vi "pulses2commands.vi"(4 "N_pulses":i32=1 min=1, 6 "running_mode":enum16{"Continuous", "Single", "N pulses"}(ring), 8 "read_width_us":dbl=0.3, 9 "read_delay_us":dbl, 10 "pulse_width_us":dbl=50.0 format="%#.3f", 11 "pulse_period_us":dbl=100.0 format="%#_6p") -> (0 "error_out":errorcluster, 3 "instructions_array":T1(array[cluster]) {"Time" format="%#_6e"})   [LabVIEW 2018]
panel:
  # "Laser Pulse"
  # "Counting pulse"
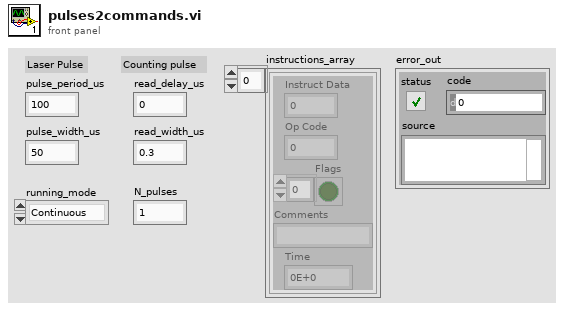
[diagram p1: front panel]
types:
  T1 = cluster{"Instruct Data":i32, "Op Code":i32, "Flags":bool[], "Comments":string, "Time":dbl}[]
  T2 = cluster{"Instruct Data":i32, "Op Code":i32, "Flags":bool[], "Comments":string, "Time":dbl}
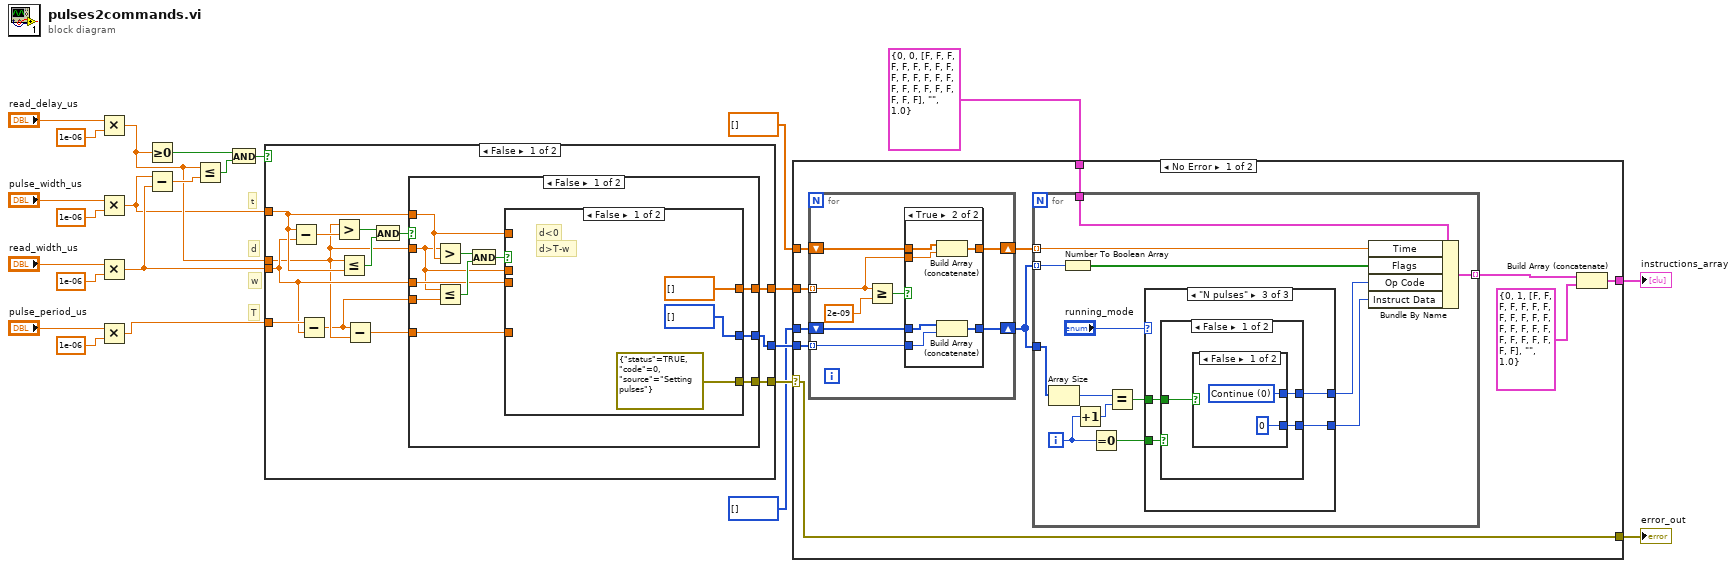
[diagram p0: block diagram]
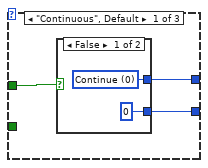
[diagram p2: hidden frame]
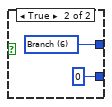
[diagram p3: hidden frame]
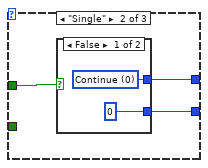
[diagram p4: hidden frame]
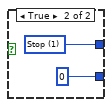
[diagram p5: hidden frame]
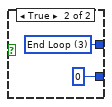
[diagram p6: hidden frame]
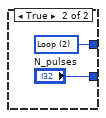
[diagram p7: hidden frame]
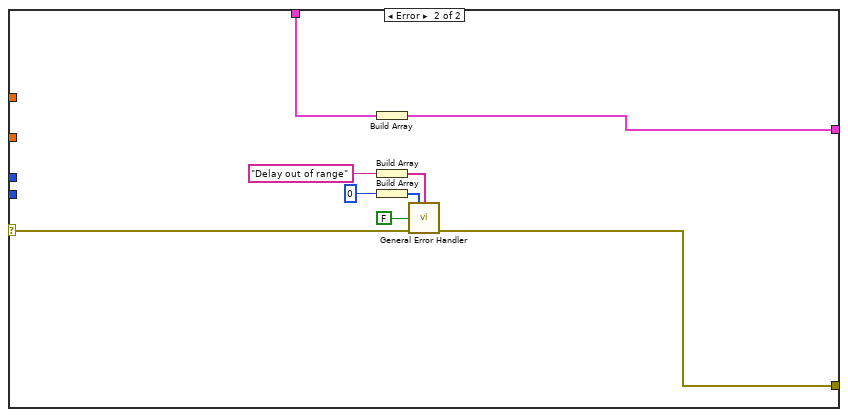
[diagram p9: hidden frame]
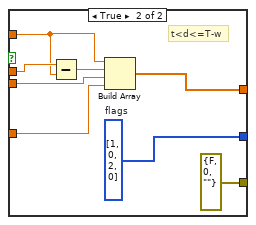
[diagram p10: hidden frame]
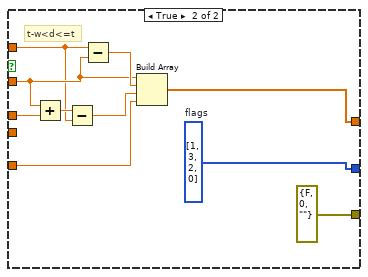
[diagram p11: hidden frame]
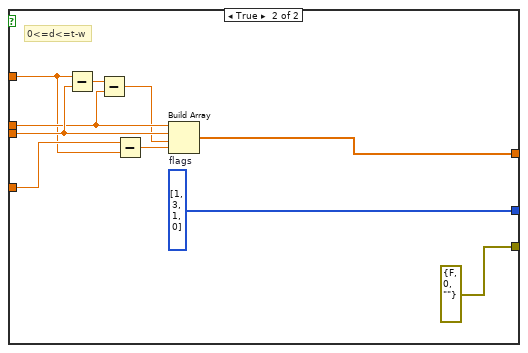
[diagram p12: hidden frame]
diagram:
  # "T"
  # "d"
  # "w"
  # "t"
  n1 = Multiply(x="read_delay_us", y=1e-06) -> (x*y=w12:dbl)
  n2 = Multiply(x="pulse_width_us", y=1e-06) -> (x*y=w4:dbl)
  n3 = Multiply(x="read_width_us", y=1e-06) -> (x*y=w16:dbl)
  n4 = Multiply(x="pulse_period_us", y=1e-06) -> (x*y=w1:dbl)
  n5 = Greater Or Equal To 0?(x=w12) -> (x >= 0?=w22:bool)
  n6 = Subtract(x=w4, y=w16) -> (x-y=w24:dbl)
  n7 = Less Or Equal?(x=w12, y=w24) -> (x <= y?=w23:bool)
  n8 = And(x=w22, y=w23) -> (x .and. y?=w21:bool)
  n9 = case shown="False" w21 {
    tunnel: w12 -> [w28 w77]
    tunnel: w16 -> [w29 w78]
    tunnel: w4 -> [w32 w70]
    tunnel: w1 -> [w33 w71]
    tunnel: [w30 w74] -> w19
    tunnel: [w26 w73] -> w20
    tunnel: [w25 errorcluster {"status"=FALSE, "code"=0, "source"=""} ("error constant")] -> w18
    frame False {
      n10 = Subtract(x=w32, y=w29) -> (x-y=w37:dbl)
      n11 = Subtract(x=w33, y=w29) -> (x-y=w27:dbl)
      n12 = Greater?(x=w28, y=w37) -> (0:w35:bool)
      n13 = Less Or Equal?(x=w28, y=w32) -> (x <= y?=w36:bool)
      n14 = Subtract(x=w27, y=w28) -> (x-y=w31:dbl)
      n15 = And(x=w35, y=w36) -> (x .and. y?=w34:bool)
      n16 = case shown="False" w34 {
        tunnel: w28 -> [w41 w68]
        tunnel: w32 -> [w44 w65]
        tunnel: w29 -> [w42 w67]
        tunnel: w31 -> [w43 w63]
        tunnel: [w40 w62] -> w30
        tunnel: w27 -> [w48 _]
        tunnel: [w39 w61] -> w26
        tunnel: [w38 errorcluster {"status"=FALSE, "code"=0, "source"=""} ("error constant")] -> w25
        frame False {
          n17 = Greater?(x=w41, y=w44) -> (0:w46:bool)
          n18 = Less Or Equal?(x=w41, y=w48) -> (x <= y?=w47:bool)
          n19 = And(x=w46, y=w47) -> (x .and. y?=w45:bool)
          n20 = case shown="False" w45 {
            tunnel: w44 -> [_ w55]
            tunnel: w43 -> [_ w59]
            tunnel: w42 -> [_ w58]
            tunnel: w41 -> [_ w56]
            tunnel: [dbl[] [] w54] -> w40
            tunnel: [u8[] [] ("flags") w53] -> w39
            tunnel: [errorcluster {"status"=TRUE, "code"=0, "source"="Setting pulses"} ("error constant") errorcluster {"status"=FALSE, "code"=0, "source"=""} ("error constant")] -> w38
            frame False {
              # "d>T-w"
              # "d<0"
            }
            frame True {
              w53 = u8[] [1, 0, 2, 0]  # flags
              # "t<d<=T-w"
              n21 = Subtract(x=w56, y=w55) -> (x-y=w57:dbl)
              n22 = Build Array(w55, w57, w58, w59) -> (w54:dbl[])
            }
          }
        }
        frame True {
          w61 = u8[] [1, 3, 2, 0]  # flags
          # "t-w<d<=t"
          n23 = Add(x=w68, y=w67) -> (x+y=w66:dbl)
          n24 = Subtract(x=w66, y=w65) -> (x-y=w64:dbl)
          n25 = Subtract(x=w65, y=w68) -> (x-y=w69:dbl)
          n26 = Build Array(w68, w69, w64, w63) -> (w62:dbl[])
        }
      }
    }
    frame True {
      w73 = u8[] [1, 3, 1, 0]  # flags
      # "0<=d<=t-w"
      n27 = Subtract(x=w70, y=w78) -> (x-y=w79:dbl)
      n28 = Subtract(x=w79, y=w77) -> (x-y=w76:dbl)
      n29 = Subtract(x=w71, y=w70) -> (x-y=w75:dbl)
      n30 = Build Array(w77, w78, w76, w75) -> (w74:dbl[])
    }
  }
  n31 = case shown="No Error" w18 {
    selector: w18 -> [w86 w154]
    tunnel: w20 -> [w84 _]
    tunnel: w19 -> [w88 _]
    tunnel: [w81 w156] -> w11
    tunnel: T2 {"Instruct Data"=0, "Op Code"=0, "Flags"=[FALSE, FALSE, FALSE, FALSE, FALSE, FALSE, FALSE, FALSE, FALSE, FALSE, FALSE, FALSE, FALSE, FALSE, FALSE, FALSE, FALSE, FALSE, FALSE, FALSE, FALSE, FALSE, FALSE, FALSE], "Comments"="", "Time"=1.0} ("PB Instruction") -> [w87 w155]
    tunnel: [w86 w153] -> w9
    tunnel: dbl[] [] ("appended array") -> [w85 _]
    tunnel: u8[] [] ("appended array") -> [w83 _]
    frame No Error {
      n32 = for {
        shift-right: [w136] -> w89
        shift-left: w83 -> [w138]
        shift-right: [w137] -> w90
        shift-left: w85 -> [w139]
        tunnel: w88 -> [w133] mode=indexing
        tunnel: w84 -> [w132] mode=indexing
        n33 = Greater Or Equal?(x=w133, y=2e-09) -> (x >= y?=w135:bool)
        n34 = case shown="True" w135 {
          tunnel: w139 -> [w140 w147]
          tunnel: w138 -> [w141 w143]
          tunnel: [w140 w146] -> w137
          tunnel: [w141 w144] -> w136
          tunnel: w133 -> [_ w145]
          tunnel: w132 -> [_ w142]
          frame False {
          }
          frame True {
            n35 = Build Array (concatenate)(w147, w145) -> (w146:dbl[])
            n36 = Build Array (concatenate)(w143, w142) -> (w144:u8[])
          }
        }
      }
      n37 = for {
        tunnel: w90 -> [w104] mode=indexing
        tunnel: w89 -> [w103] mode=indexing
        tunnel: [w97] -> w82 mode=indexing
        tunnel: w89 -> [w98]
        tunnel: w87 -> [w101]
        i -> [w95]
        n38 = Array Size(array=w98) -> (size(s)=w99:i32)
        n39 = Number To Boolean Array(number=w103) -> (Boolean array=w102:bool[])
        n40 = Increment(x=w95) -> (x+1=w100:i32)
        n41 = Equal To 0?(x=w95) -> (x = 0?=w93:bool)
        n42 = Equal?(x=w99, y=w100) -> (x = y?=w94:bool)
        n43 = case shown="\"N pulses\"" "running_mode" {
          tunnel: w94 -> [w105 w112 w122]
          tunnel: [w107 w114 w121] -> w92
          tunnel: [w106 w113 w120] -> w91
          tunnel: w93 -> [_ _ w119]
          frame "Continuous", Default {
            n44 = case shown="False" w105 {
              tunnel: [w109 w111] -> w107
              tunnel: [0 ("N_pulses") 0 ("N_pulses")] -> w106
              frame False {
                w109 = 0 items=["Continue", "Stop", "Loop", "End Loop", "JSR", "RTS", "Branch", "Long Delay", "Wait"] ("Op Code")
              }
              frame True {
                w111 = 6 items=["Continue", "Stop", "Loop", "End Loop", "JSR", "RTS", "Branch", "Long Delay", "Wait"] ("Op Code")
              }
            }
          }
          frame "Single" {
            n45 = case shown="False" w112 {
              tunnel: [w116 w118] -> w114
              tunnel: [0 ("N_pulses") 0 ("N_pulses")] -> w113
              frame False {
                w116 = 0 items=["Continue", "Stop", "Loop", "End Loop", "JSR", "RTS", "Branch", "Long Delay", "Wait"] ("Op Code")
              }
              frame True {
                w118 = 1 items=["Continue", "Stop", "Loop", "End Loop", "JSR", "RTS", "Branch", "Long Delay", "Wait"] ("Op Code")
              }
            }
          }
          frame "N pulses" {
            n46 = case shown="False" w119 {
              tunnel: w122 -> [w123 _]
              tunnel: [w125 w131] -> w121
              tunnel: [w124 "N_pulses"] -> w120
              frame False {
                n47 = case shown="False" w123 {
                  tunnel: [w127 w129] -> w125
                  tunnel: [0 ("N_pulses") 0 ("N_pulses")] -> w124
                  frame False {
                    w127 = 0 items=["Continue", "Stop", "Loop", "End Loop", "JSR", "RTS", "Branch", "Long Delay", "Wait"] ("Op Code")
                  }
                  frame True {
                    w129 = 3 items=["Continue", "Stop", "Loop", "End Loop", "JSR", "RTS", "Branch", "Long Delay", "Wait"] ("Op Code")
                  }
                }
              }
              frame True {
                w131 = 2 items=["Continue", "Stop", "Loop", "End Loop", "JSR", "RTS", "Branch", "Long Delay", "Wait"] ("Op Code")
              }
            }
          }
        }
        n48 = Bundle By Name(cluster=w101, "Time"=w104, "Flags"=w102, "Op Code"=w92, "Instruct Data"=w91) -> (w97:T2)
      }
      n49 = Build Array (concatenate)(w82, T2 {"Instruct Data"=0, "Op Code"=1, "Flags"=[FALSE, FALSE, FALSE, FALSE, FALSE, FALSE, FALSE, FALSE, FALSE, FALSE, FALSE, FALSE, FALSE, FALSE, FALSE, FALSE, FALSE, FALSE, FALSE, FALSE, FALSE, FALSE, FALSE, FALSE], "Comments"="", "Time"=1.0} ("PB Instruction")) -> (w81:T1)
    }
    frame Error {
      n50 = Build Array(w155) -> (w156:T1)
      n51 = Build Array("Delay out of range") -> (w150:string[])
      n52 = Build Array(0) -> (w148:i32[])
      n53 = call <vilib>:"General Error Handler.vi"("[user-defined codes]"=w148, "[user-defined descriptions]"=w150, "search ni.com link visible?(T)"=FALSE, "error in (no error)"=w154) -> ("error out"=w153:errorcluster)  [unwired: 7 in, 4 out]
    }
  }
  "instructions_array" <- w11
  "error_out" <- w9
